vi "Write pauseStartTime.vi"(10 "pauseStartTime":timestamp, 11 "TestMonitor in":refnum<class "TestMonitor.lvclass">) -> (3 "TestMonitor out":refnum<class "TestMonitor.lvclass">)   [LabVIEW 2013, in "TestMonitor.lvclass"]
uses:
  TestMonitor.lvclass
  TestMonitor.lvclass/TestMonitor.ctl
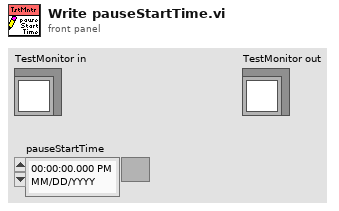
[diagram p1: front panel]
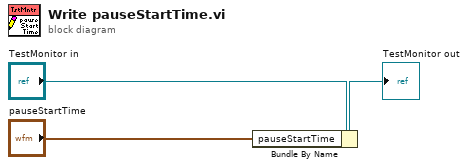
[diagram p0: block diagram]
diagram:
  n1 = Bundle By Name(cluster="TestMonitor in", "pauseStartTime"="pauseStartTime") -> (→"TestMonitor out":refnum<class "TestMonitor.lvclass">)
